vi "SingleServiceRegistered_InvalidResolveRequests_Error.vi"() -> (6 "pass":bool, 8 "result":string, 15 "error out":errorcluster)   [LabVIEW 2020]
uses:
  Discovery Client_lv/Discovery_client/RPC Messages/ni_measurementlink_discovery_v1_RegisterServiceRequest.ctl
  Discovery Client_lv/Discovery_client/RPC Messages/ni_measurementlink_discovery_v1_ServiceDescriptor.ctl
  Discovery Client_lv/Discovery_client/RPC Messages/ni_measurementlink_discovery_v1_ServiceLocation.ctl
  Discovery Client_lv/Discovery_client/RPC Messages/ni_measurementlink_discovery_v1_ResolveServiceRequest.ctl
  Discovery Client_lv/Discovery_client/Discovery_client.lvlib
panel:
  # "Test assumes discovery service has already been started."
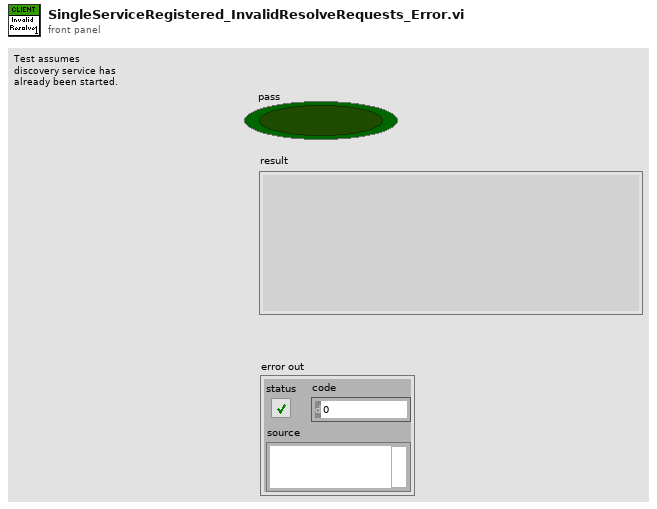
[diagram p1: front panel]
types:
  T1 = typedef "Discovery_client.lvlib/ni_measurementlink_discovery_v1_ResolveServiceRequest.ctl" = cluster{"provided_interface":string, "service_class":string}
  T2 = typedef "Discovery_client.lvlib/ni_measurementlink_discovery_v1_RegisterServiceRequest.ctl" = cluster{"service_description":T3, "location":T4}
  T3 = typedef "Discovery_client.lvlib/ni_measurementlink_discovery_v1_ServiceDescriptor.ctl" = cluster{"display_name":string, "description_url":string, "provided_interfaces":string[], "service_class":string, "attributes":string[]}
  T4 = typedef "Discovery_client.lvlib/ni_measurementlink_discovery_v1_ServiceLocation.ctl" = cluster{"location":string, "insecure_port":string, "ssl_authenticated_port":string}
  T5 = typedef "Discovery_client.lvlib/ni_measurementlink_discovery_v1_RegisterServiceResponse.ctl" = cluster{"registration_id":string}
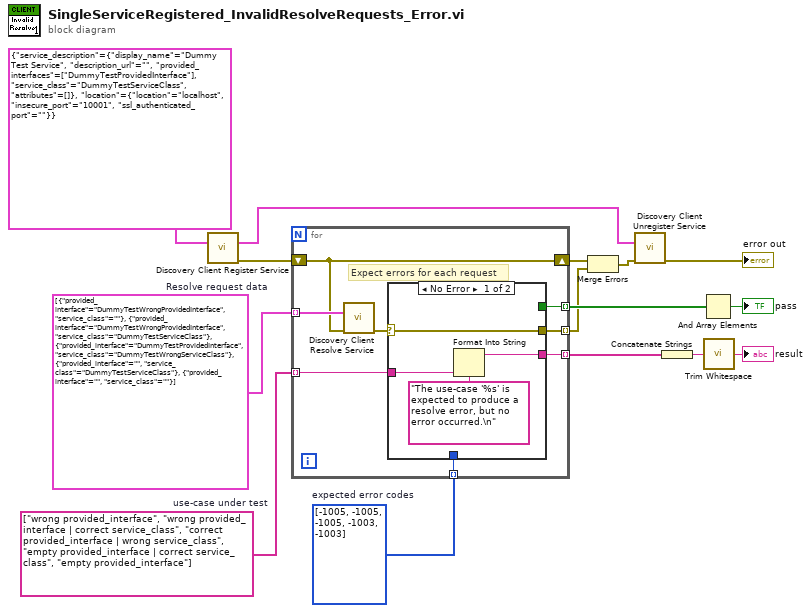
[diagram p0: block diagram]
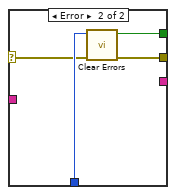
[diagram p2: hidden frame]
diagram:
  w2 = string[] ["wrong provided_interface", "wrong provided_interface | correct service_class", "correct provided_interface | wrong service_class", "empty provided_interface | correct service_class", "empty provided_interface"]  # use-case under test
  w8 = i32[] [-1005, -1005, -1005, -1003, -1003]  # expected error codes
  w11 = T1[] [{"provided_interface"="DummyTestWrongProvidedInterface", "service_class"=""}, {"provided_interface"="DummyTestWrongProvidedInterface", "service_class"="DummyTestServiceClass"}, {"provided_interface"="DummyTestProvidedInterface", "service_class"="DummyTestWrongServiceClass"}, {"provided_interface"="", "service_class"="DummyTestServiceClass"}, {"provided_interface"="", "service_class"=""}]  # Resolve request data
  n1 = call "Discovery Client Register Service.vi"("Request Data"=T2 {"service_description"={"display_name"="Dummy Test Service", "description_url"="", "provided_interfaces"=["DummyTestProvidedInterface"], "service_class"="DummyTestServiceClass", "attributes"=[]}, "location"={"location"="localhost", "insecure_port"="10001", "ssl_authenticated_port"=""}}) -> ("Response Data"=w15:T5, "error out"=w13:errorcluster)  [unwired: 13 in]
  n2 = for {
    tunnel: w11 -> [w23] mode=indexing
    shift-right: [w22] -> w7
    shift-left: w13 -> [w22]
    tunnel: [w18] -> w9 mode=indexing
    tunnel: w8 -> [w20] mode=indexing
    tunnel: [w19] -> w5 mode=indexing
    tunnel: w2 -> [w17] mode=indexing
    tunnel: [w16] -> w1 mode=indexing
    # "Expect errors for each request"
    n3 = call "Discovery Client Resolve Service.vi"("Request Data"=w23, "error in (no error)"=w22) -> ("error out"=w21:errorcluster)  [unwired: 12 in, 1 out]
    n4 = case shown="No Error" w21 {
      selector: w21 -> [w27 w28]
      tunnel: [_ w31] -> w18
      tunnel: [w27 w30] -> w19
      tunnel: w20 -> [_ w29]
      tunnel: w17 -> [w25 _]
      tunnel: [w24 _] -> w16
      frame No Error {
        n5 = Format Into String(format string="The use-case '%s' is expected to produce a resolve error, but no error occurred.\n", w25) -> (resulting string=w24:string)  [unwired: 2 in, 1 out]
      }
      frame Error {
        n6 = call <vilib>:"Clear Errors.vi"("error in (no error)"=w28, "specific error code to clear (0: all)"=w29) -> ("error out"=w30:errorcluster, "specific error cleared?"=w31:bool)  [unwired: 4 in]
      }
    }
  }
  n7 = Merge Errors(w7, w5) -> (w6:errorcluster)
  n8 = call "Discovery Client Unregister Service.vi"("Request Data"=w15, "error in (no error)"=w6) -> ("error out"=→"error out":errorcluster)  [unwired: 12 in, 1 out]
  n9 = Concatenate Strings(w1) -> (w4:string)
  n10 = And Array Elements(Boolean array=w9) -> (logical AND=→"pass":bool)
  n11 = call <vilib>:"Trim Whitespace.vi"("string"=w4) -> ("trimmed string"=→"result":string)  [unwired: 1 in]
